vi "Rack-Start.vi"(8 "error in (no error)":errorcluster, 10 "OutputRequest event ref":T1, 11 "Configuration":T2={"DigitalInput"={"Lines"=["6289/port1/line0", "6289/port1/line1", "6289/port1/line2", "6289/port1/line3"], "Refresh period (ms)"=2}, "DigitalOutput"={"Output Lines"=["6289/port0/line1", "6289/port0/line2", "6289/port0/line3"], "DO timestamp lines"=["6289/port0/line1", "6289/port0/line2", "6289/port0/line3", "6289/port0/line4", "6289/port0/line5", "6289/port0/line6", "6289/port0/line7"], "Timestamp lines"=[]}, "FileOutput"={"Logfile path"=path "C:/Users/kevin/Desktop/lvlog.txt"}, "AnalogOutput"={"Output Lines"=["6289/port0/line1", "6289/port0/line2", "6289/port0/line3", "6289/port0/line4", "6289/port0/line5", "6289/port0/line6", "6289/port0/line7"], "AO timestamp lines"=["6289/port0/line1", "6289/port0/line2", "6289/port0/line3", "6289/port0/line4", "6289/port0/line5", "6289/port0/line6", "6289/port0/line7"]}, "DataSocketOutput"={"DataSocket URL"=""}}) -> (0 "error out":errorcluster, 2 "OutputRequest event ref (dup)":T1)   [LabVIEW 2015]
doc: "Starts the rack drivers running.\n\nConfiguration: config cluster from Rack-Config.\nOutputRequest event ref: User Event refnum for communicating with the output drivers.\n\nThe output connection is just a duplicate of OutputRequest event ref to assist you in laying out your Main VI"
uses:
  Typedefs/OutputRequest refnum.ctl
  Typedefs/OutputRequest.ctl
  Typedefs/Rack driver configuration cluster.ctl
  Port drivers/DigitalInput-Configuration.ctl
  Port drivers/DigitalOutput-Configuration.ctl
  Port drivers/FileOutput-Configuration.ctl
  Port drivers/AnalogOutput-Configuration.ctl
  Port drivers/DataSocketOutput-Configuration.ctl
panel:
  # "Timestamp lines must be on an M-Series card (i.e. NOT the 6509)"
  # "Timestamp lines must be on same device as its corresponding DO line"
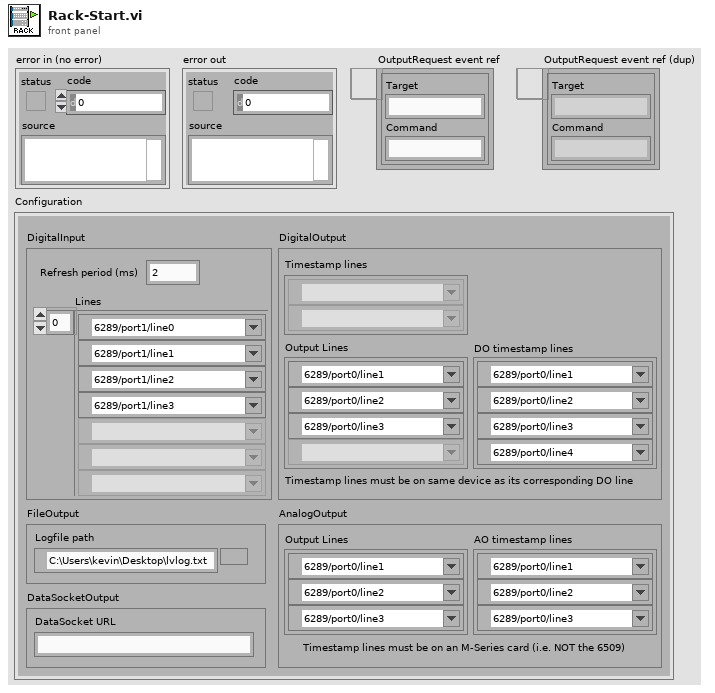
[diagram p1: front panel]
types:
  T1 = typedef "OutputRequest refnum.ctl" = refnum<user-event>
  T2 = typedef "Rack driver configuration cluster.ctl" = cluster{"DigitalInput":T3, "DigitalOutput":T4, "FileOutput":T5, "AnalogOutput":T6, "DataSocketOutput":T7}
  T3 = typedef "DigitalInput-Configuration.ctl" = cluster{"Lines":tag[], "Refresh period (ms)":u32}
  T4 = typedef "DigitalOutput-Configuration.ctl" = cluster{"Output Lines":tag[], "DO timestamp lines":tag[], "Timestamp lines":tag[]}
  T5 = typedef "FileOutput-Configuration.ctl" = cluster{"Logfile path":path}
  T6 = typedef "AnalogOutput-Configuration.ctl" = cluster{"Output Lines":tag[], "AO timestamp lines":tag[]}
  T7 = typedef "DataSocketOutput-Configuration.ctl" = cluster{"DataSocket URL":string}
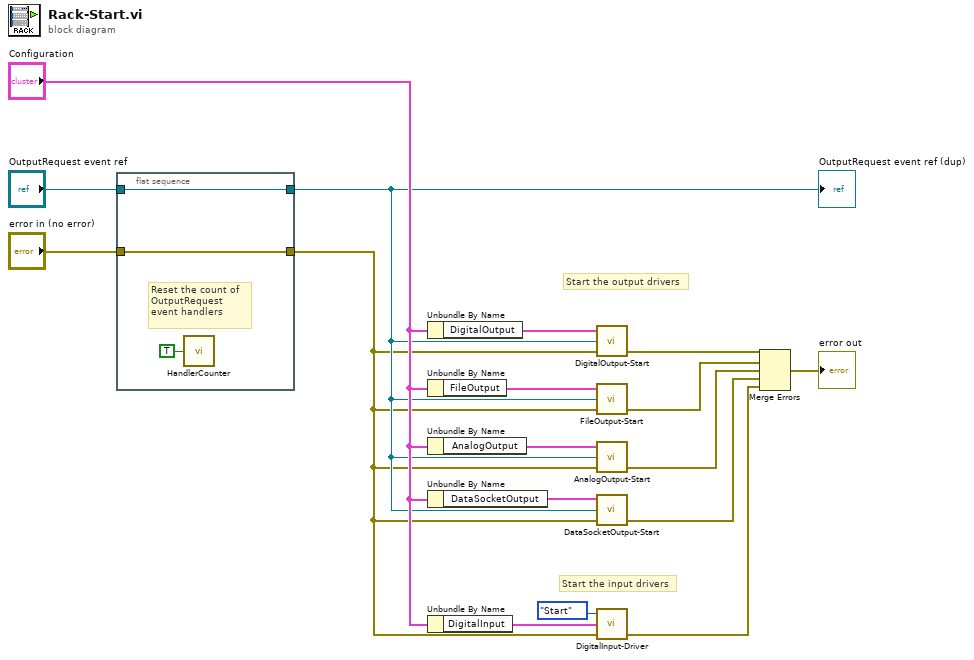
[diagram p0: block diagram]
diagram:
  # "Start the input drivers"
  # "Start the output drivers"
  n1 = flat-sequence {
    tunnel: "error in (no error)" -> [w18]
    tunnel: [w18] -> w3
    tunnel: [w19] -> w4
    tunnel: "OutputRequest event ref" -> [w19]
    frame #0 {
      # "Reset the count of \nOutputRequest\nevent handlers"
      n2 = call "HandlerCounter.vi"("Reset Count"=TRUE) -> ()  [unwired: 3 in, 2 out]
    }
  }
  n3 = Unbundle By Name("Configuration") -> ("DigitalOutput"=w10:T4)
  n4 = Unbundle By Name("Configuration") -> ("FileOutput"=w9:T5)
  n5 = Unbundle By Name("Configuration") -> ("AnalogOutput"=w8:T6)
  n6 = Unbundle By Name("Configuration") -> ("DataSocketOutput"=w6:T7)
  n7 = Unbundle By Name("Configuration") -> ("DigitalInput"=w7:T3)
  n8 = call "DigitalOutput-Start.vi"("error in (no error)"=w3, "OutputRequest\nuser event refnum"=w4, "Configuration"=w10) -> ("error out"=w15:errorcluster)  [unwired: 2 in]
  n9 = call "FileOutput-Start.vi"("error in (no error)"=w3, "OutputRequest\nuser event refnum"=w4, "Configuration"=w9) -> ("error out"=w13:errorcluster)  [unwired: 2 in]
  n10 = call "AnalogOutput-Start.vi"("error in (no error)"=w3, "OutputRequest\nuser event refnum"=w4, "Configuration"=w8) -> ("error out"=w11:errorcluster)  [unwired: 2 in]
  n11 = call "DataSocketOutput-Start.vi"("error in (no error)"=w3, "OutputRequest\nuser event refnum"=w4, "Configuration"=w6) -> ("error out"=w1:errorcluster)  [unwired: 2 in]
  n12 = call "DigitalInput-Driver.vi"("error in (no error)"=w3, "Configuration"=w7, "Command"=enum16{"Refresh", "Start", "Stop"}."Start") -> ("error out"=w2:errorcluster)  [unwired: 1 in, 1 out]
  n13 = Merge Errors(w15, w13, w11, w1, w2) -> (→"error out":errorcluster)
  "OutputRequest event ref (dup)" <- w4
